vi "Wait_for_stable_pressure.vi"() -> (0 "Aborted?":bool, 1 "Pressure Stable?":bool)   [LabVIEW 2016]
uses:
  Globals/PressuresGlobal.vi
panel:
  in  "Cancel Button":bool
  out "Waiting for stable pressure":u8(slide) scale=0.0..100.0
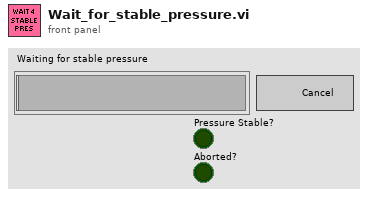
[diagram p1: front panel]
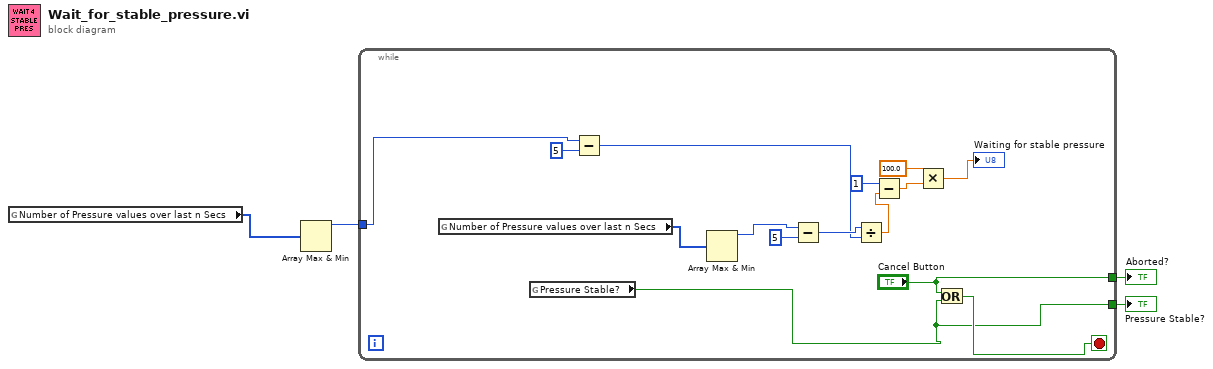
[diagram p0: block diagram]
diagram:
  n1 = global read "PressuresGlobal.vi" "Number of Pressure values over last n Secs"() -> (w4:i32[])
  n2 = Array Max & Min(array=w4) -> (max value=w3:i32)  [unwired: 3 out]
  n3 = while {
    tunnel: [w18] -> w2
    tunnel: ["Cancel Button"] -> w1
    tunnel: w3 -> [w14]
    stop <- w19 stop-if-true
    n4 = global read "PressuresGlobal.vi" "Number of Pressure values over last n Secs"() -> (w16:i32[])
    n5 = global read "PressuresGlobal.vi" "Pressure Stable?"() -> (w18:bool)
    n6 = Subtract(x=w14, y=u8 5) -> (x-y=w10:i32)
    n7 = Array Max & Min(array=w16) -> (max value=w12:i32)  [unwired: 3 out]
    n8 = Subtract(x=w12, y=u8 5) -> (x-y=w11:i32)
    n9 = Divide(x=w11, y=w10) -> (x/y=w8:dbl)
    n10 = Subtract(x=i8 1, y=w8) -> (x-y=w7:dbl)
    n11 = Multiply(x=100.0, y=w7) -> (x*y=→"Waiting for stable pressure":dbl)
    n12 = Or(x="Cancel Button", y=w18) -> (x .or. y?=w19:bool)
  }
  "Pressure Stable?" <- w2
  "Aborted?" <- w1
